vi "EnqueueMultipleAutoMode.vi"(6 "Priority Message":bool, 8 "error in (no error)":errorcluster, 9 "Data":variant[](array[variant]), 10 "AutoState":T1[](array[typedef]), 11 "Queue in":refnum<queue>) -> (0 "error out":errorcluster, 3 "queue out":refnum<queue>)   [LabVIEW 2019, in "AutoMode.lvlib"]
uses:
  AutoMode.lvlib
  Enum - AutoModeState.ctl
  Cluster - AutoModeMessage.ctl
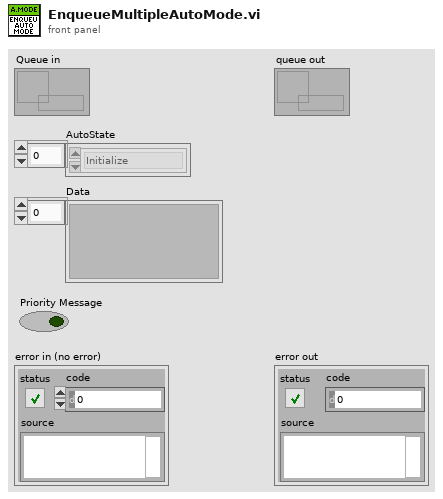
[diagram p1: front panel]
types:
  T1 = typedef "AutoMode.lvlib/Enum - AutoModeState.ctl" = enum16{"Initialize", "Idle", "UpdateConfig", "UpdateHWConfig", "BroadcastSettings", "Start", "CheckValidReportPath", "Winding", "WaitForWinding", "Unwind", "WaitForUnwind", "Stop", "Abort", "WriteDataToFile", "EventTriggered", "GenerateFilePath", "ZeroPosition", "GotoZero", "Error", "Exit"}
  T2 = typedef "AutoMode.lvlib/Cluster - AutoModeMessage.ctl" = cluster{"Message":T1, "Data":variant}
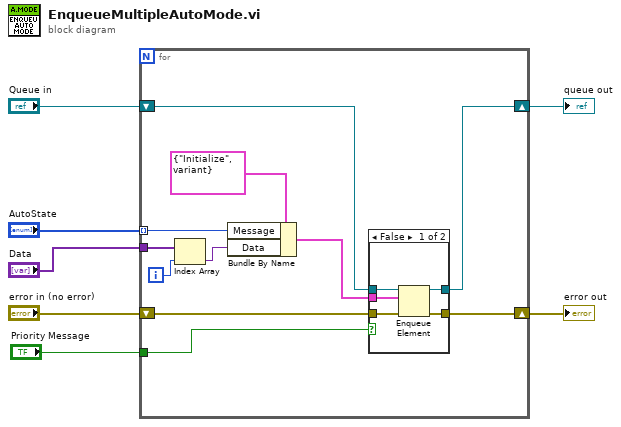
[diagram p0: block diagram]
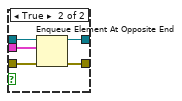
[diagram p2: hidden frame]
diagram:
  n1 = for {
    tunnel: "AutoState" -> [w15] mode=indexing
    tunnel: "Data" -> [w14]
    tunnel: "Priority Message" -> [w10]
    shift-right: [w18] -> w7
    shift-left: "error in (no error)" -> [w13]
    shift-right: [w11] -> w2
    shift-left: "Queue in" -> [w12]
    i -> [w8]
    n2 = Index Array(array=w14, index=w8) -> (element=w9:variant)
    n3 = Bundle By Name(cluster=T2 {"Message"=enum."Initialize", "Data"=variant} ("CycleTestMessage"), "Message"=w15, "Data"=w9) -> (w16:T2)
    n4 = case shown="False" w10 {
      tunnel: [w22 w28] -> w18
      tunnel: w16 -> [w19 w27]
      tunnel: w13 -> [w23 w26]
      tunnel: w12 -> [w21 w25]
      tunnel: [w20 w24] -> w11
      frame False {
        n5 = Enqueue Element(queue=w21, element=w19, error in (no error)=w23) -> (queue out=w20:refnum<queue>, error out=w22:errorcluster)  [unwired: 1 in, 1 out]
      }
      frame True {
        n6 = Enqueue Element At Opposite End(queue=w25, element=w27, error in (no error)=w26) -> (queue out=w24:refnum<queue>, error out=w28:errorcluster)  [unwired: 1 in, 1 out]
      }
    }
  }
  "error out" <- w7
  "queue out" <- w2
